vi "Dropable_DSA.vi"(0 "Analog In CH1":dbl, 1 "Cycle Specs":T3={"Cycles To Settle (M)"=5, "Cycles To Calculate (N)"=5}, 2 "Excitation Specs":T2={"Initial Frequency"=1.0, "Final Frequency"=100.0, "# of pts. in interval"=3, "Samping Time [s]"=0.001, "Amplitude [V]"=1.0, "Offset [V]"=0.5, "Freq Units (F: rad/s, T: Hz)"=FALSE}, 5 "Analog In CH0":dbl, 9 "START":bool, 11 "STOP":bool, 12 "Exit Porgram":bool) -> (4 "Analog Out":dbl, 6 "Bode Magnitude":cluster{dbl[], dbl[]}(graph)={[1.0, 1.2689610031679222, 1.6102620275609394, 2.043359717856942, 2.592943797404667, 3.2903445623126686, 4.1753189365604015, 5.298316906283708, 6.7233575364993365, 8.531678524172808, 10.826367338740546, 13.73823795883263, 17.43328822199988, 22.122162910704493, 28.072162039411772, 35.62247890262442, 45.20353656360243, 57.36152510448679, 72.7895384398315, 92.36708571873861, 117.21022975334806, 148.73521072935117, 188.73918221350976, 239.5026619987486, 303.9195382313198, 385.6620421163472, 489.3900918477494, 621.0169418915616, 788.0462815669912, 1000.0], [1.0018651131002922, 1.0016050465725763, 1.0010062349698785, 1.0002931137870483, 0.9991459144089636, 0.9972202532472595, 0.9944020144562293, 0.9903082002861369, 0.983855401702225, 0.9738705481650444, 0.9582906977613652, 0.9358034848813956, 0.9036393454169751, 0.857649976648417, 0.7964400088413218, 0.7217565791716765, 0.6359239660806931, 0.5476382842843324, 0.461415834347026, 0.38116988425483045, 0.3091314427820101, 0.2514928062528439, 0.20170891904461263, 0.15879614847289658, 0.127858110424497, 0.10171304349328705, 0.08081117825531599, 0.06376794604720305, 0.050469140870365095, 0.039745706120179934]}, 8 "Bode Phase":cluster{dbl[], dbl[]}(graph)={[1.0, 1.2689610031679222, 1.6102620275609394, 2.043359717856942, 2.592943797404667, 3.2903445623126686, 4.1753189365604015, 5.298316906283708, 6.7233575364993365, 8.531678524172808, 10.826367338740546, 13.73823795883263, 17.43328822199988, 22.122162910704493, 28.072162039411772, 35.62247890262442, 45.20353656360243, 57.36152510448679, 72.7895384398315, 92.36708571873861, 117.21022975334806, 148.73521072935117, 188.73918221350976, 239.5026619987486, 303.9195382313198, 385.6620421163472, 489.3900918477494, 621.0169418915616, 788.0462815669912, 1000.0], [-1.4001864556390353, -1.7425257743205063, -2.2774811113746067, -2.940300047591337, -3.797024621582645, -4.874740361894845, -6.244214499985965, -7.9488896703659435, -10.107416371370137, -12.8129960492024, -16.195047872218314, -20.2121008365249, -24.982209581081694, -30.62002310970157, -36.70295501035055, -43.18506539585506, -49.773026506300724, -56.0120451118291, -61.68921924132383, -66.61507141784128, -71.21117465500357, -75.07757805867544, -77.49128997241446, -81.82799122918105, -82.40583459630555, -84.09391534817092, -87.5421411007668, -88.23137376055858, -91.93060722680163, -98.46625820370649]}, 10 "Live signals":T1(graph), 14 "Stopped":bool, 15 "Running":bool)   [LabVIEW 2018]
doc: "Evaluate frequency response: CH1/CH0\n\nThis program performs 3 tasks:\n\n A.) generates a swept sine wave over a specified number of logmartically spaced frequencies over a specified range,\n\n B.) outputs the swept sine wave point by point to a system and for each point output measues the system's response at two points\n\n C.) and using the two responses measured, calculates the bode magnitude and phase plots between the two points of the system.\n\nThis program is written as a state machine that itterates one time for every iteration of the loop that contains it.\n \nThe state is the current sample being measured. \nNOTE: Since we must excite the system before recording data, the current sample being measured is one less than the number of itterations the loop containing this subVI has run.\n\nTo perform these tasks, the following state machine does the following:\n\n INITIALIZATION \n\n When initalized, the state is set to 0 and the following are calculated:\n\n A.) a list of logmartically spaced frequencies to excite the system at, \n B.) the number of samples needed to be ignored in waiting for the excitation to settle for each frequency, \n C.) the number of samples needed to be measured in order to calculate the frequency response for each frequency,\n D.) and the total number of samples needed (total # of smaples ignored + total # of samples measured).\n\n < see (1) INITIALIZE THE DSA section in the block diagram >\n\n RUNNING\n\n When running, the following tasks are done:\n\n A.) The swept sine wave for the next sample to be measured is generated and output. \n This is done by generating:\n\n 1.) the ith point of the swept sine wave to excite the system\n 2.) the frequency of the sine wave for the current point\n 3.) and the index of the frequency within the list excitation frequencies that corresponds to the i+1 point's sine wave's frequency.\n\n < see (2A) GENERATE SWEPT SINE EXCITATIONS section in the block diagram >\n\n B.) Compare the current sample to:\n\n 1.) the current last sample to be ignored in the list of last samples to be ignored\n 2.) and the current last smaple taken before chaning frequencies in the list of sample taken before the frequency change.\n\n < see (2B) COLLECT DATA? section in the block diagram >\n\n C.) If the current sample:\n \n 1.) < the current last sample to be ignored:\n \n - do nothing.\n \n 2.) = the current last sample to be ignored and:\n\n\n a.) < the current sample taken before changing frequencies:\n \n - collect a sample on each channel and store it\n\n < see (2C) ANALYZE DATA section in the block diagram >\n\n b.) = the current sample taken before changing frequencies:\n\n i.) collect a sample on each channel and store it,\n ii.) with all the other samples stored for that excitation frequency, calculate the magnitude and phase for each channel,\n iii.) use the magnitude and phase for each channel to calculate the magnitude and phase between the two points in the system,\n iv.) and plot the magnitude and phase between those two points in the system on the bode plot for the frequency.\n \n < see (2D) VERIFY DATA & (2E) PLOT section in the block diagram >\n\nInputs: \n\n- Excitation Specs:\n\n - Initial Frequency: The lowest frequency of the frequency range which the DSA will measure the bode plot for. \n\n - Final Frequency: The highest frequency of the frequency range which the DSA will measure the bode plot for. \n\n - Frequency Units: Whether the frequecny range input is in Hz or rads/sec. \n \n - Number of Frequencies: The number of logmarithmically spaced frequencies to measure the bode plot for.\n\n - Sampling Time: The time step taking in between each measurement. Also equal to 1/(sampling rate)\n\n - Amplitude: Amplitude of desired swept sine excitation. \n\n - Offset: DC offset of swept sine excitation.\n\n- Cycle Specs:\n\n - Cycles to Settle: The number of cycles of the swept sine wave at each frequency to ignore to let the transcient response die out. \n\n - Cycles to Calculate: The number of cycles of the sept since wave at each frequency to measure in order to measure the bode plot.\n\n- Controls:\n\n - START: Tells the DSA to initalize and then start.\n\n - STOP: Tells the DSA to stop and set all analog outputs to zero.\n\n - EXIT PROGRAM: Tells LabVIEW to set all analog outputs to zero and exit the program.\n\n- Signals:\n\n - Analog In CH1: Response read by the A/D converter of the system at a given point to the swept sine excitation.\n\n - Analog In CH0: Response read by the A/D converter of the system at a given point to the swept sine excitation.\n\nOutputs:\n\n- Analog Out: Swept sine excitation wave sent to the D/A converter.\n\n- Running: Signal to show if the DSA is running.\n\n- Stopped: Signal to show if the DSA is stopped.\n\n- Bode Magnitude: The magnitude plot of the TF CH1/CH0.\n\n- Bode Phase: The phase plot of the TF CH1/CH0."
panel:
  # "Dropable Dynamic Signal Analyzer"
  # "Magnitude"
  # "Dynamic Signal Analyzer"
  # "Controls"
  # "Signals"
  # "Phase"
  # "Excitation Frequencies"
  # "Frequency\nUnits"
  # "[Hz]"
  # "Excitation Magnitude"
  # "[rad/s]"
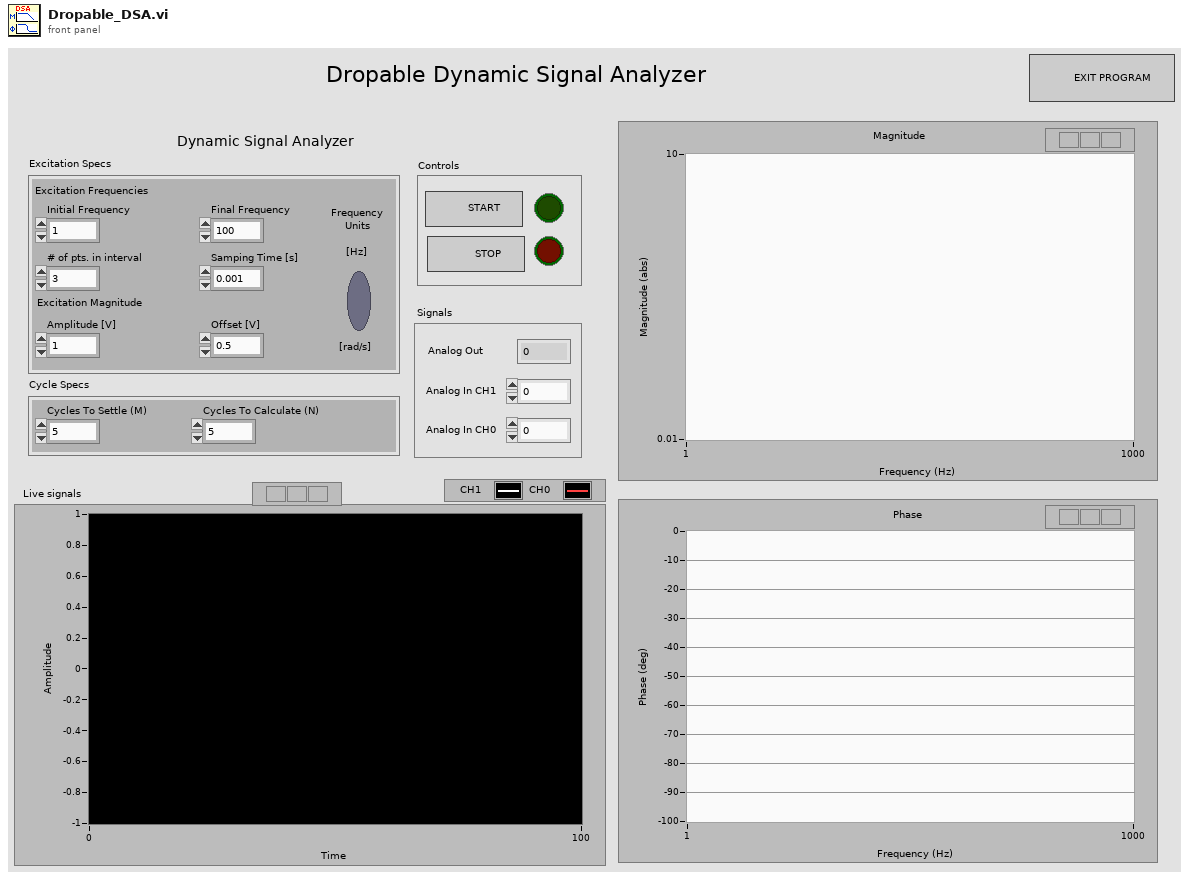
[diagram p1: front panel]
types:
  T1 = cluster{"Analog In CH1":dbl, "Analog In CH0":dbl}
  T2 = cluster{"Initial Frequency":dbl, "Final Frequency":dbl, "# of pts. in interval":i16, "Samping Time [s]":dbl, "Amplitude [V]":dbl, "Offset [V]":dbl, "Freq Units (F: rad/s, T: Hz)":bool}
  T3 = cluster{"Cycles To Settle (M)":i16, "Cycles To Calculate (N)":i16}
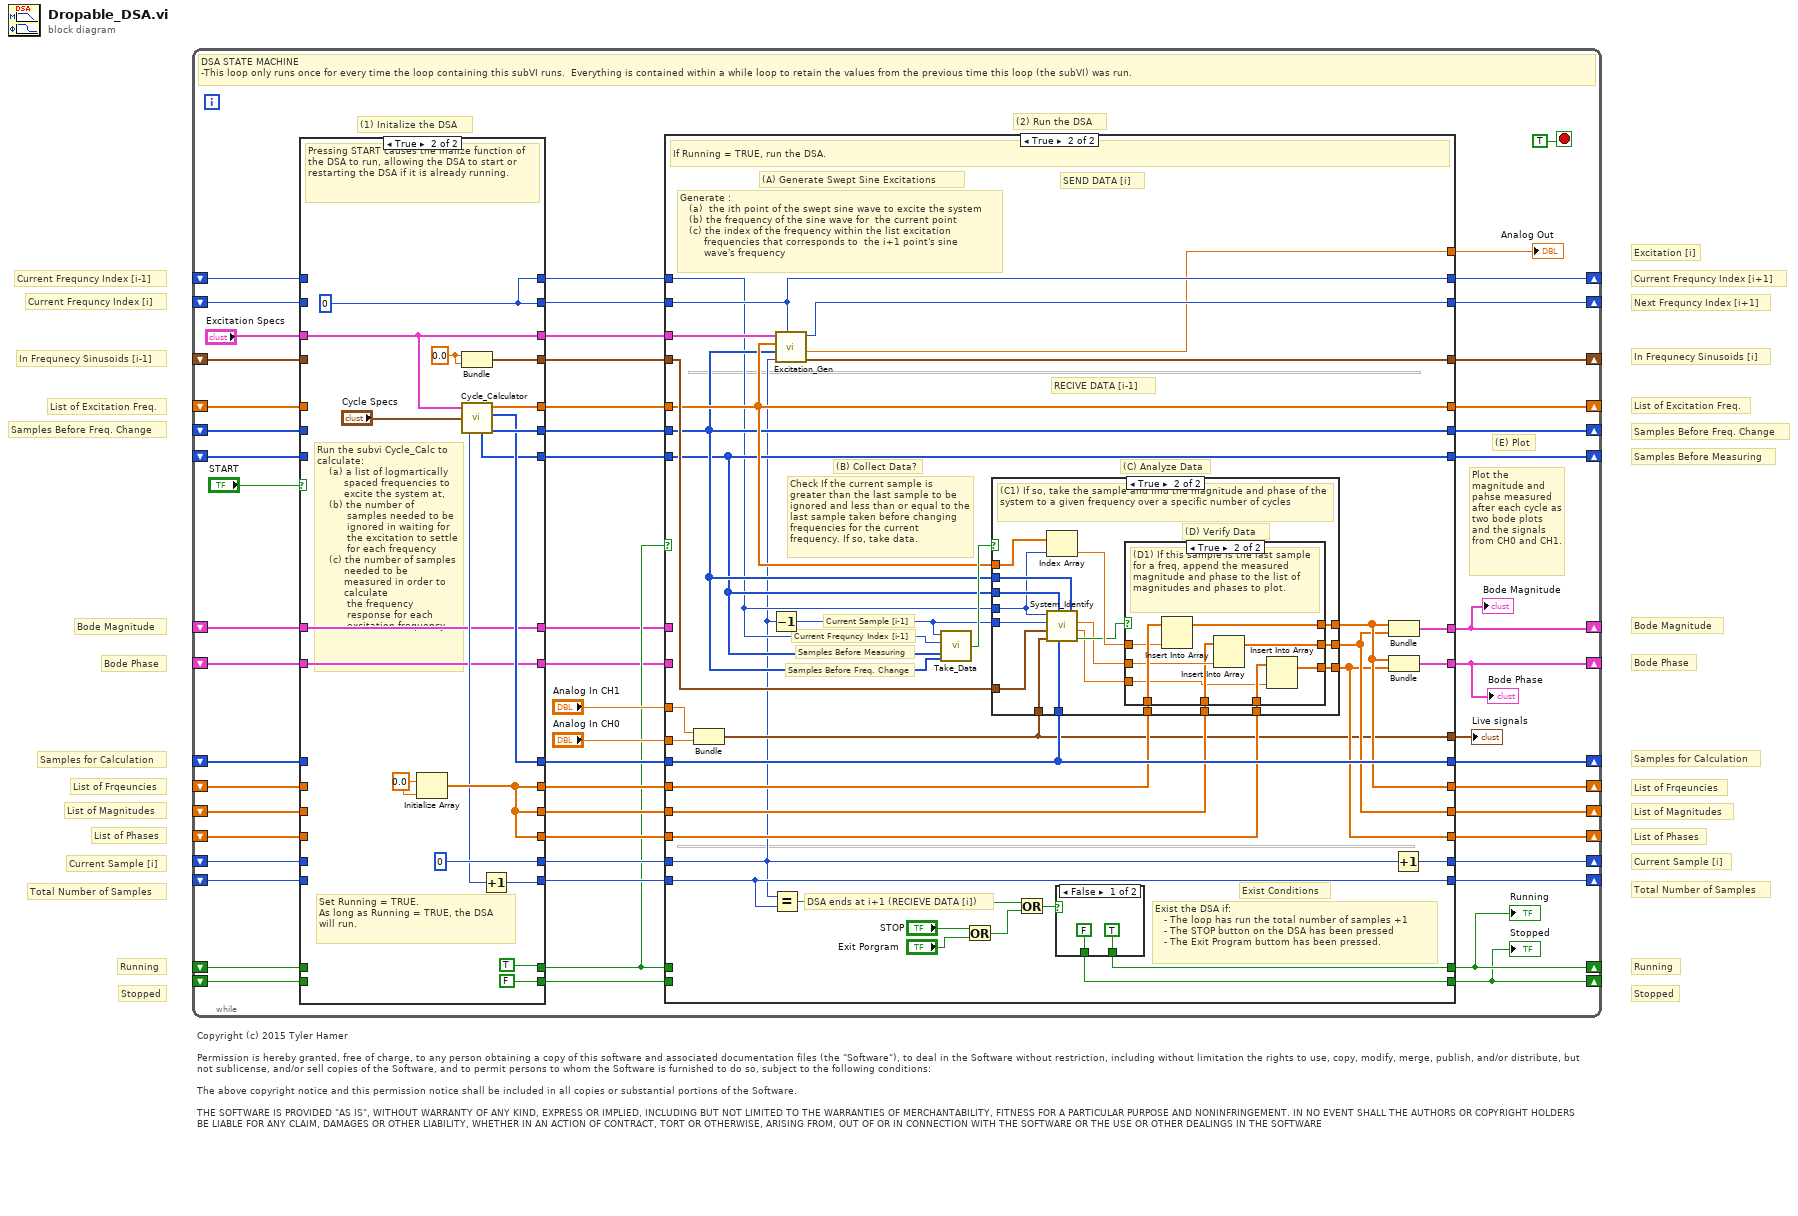
[diagram p0: block diagram]
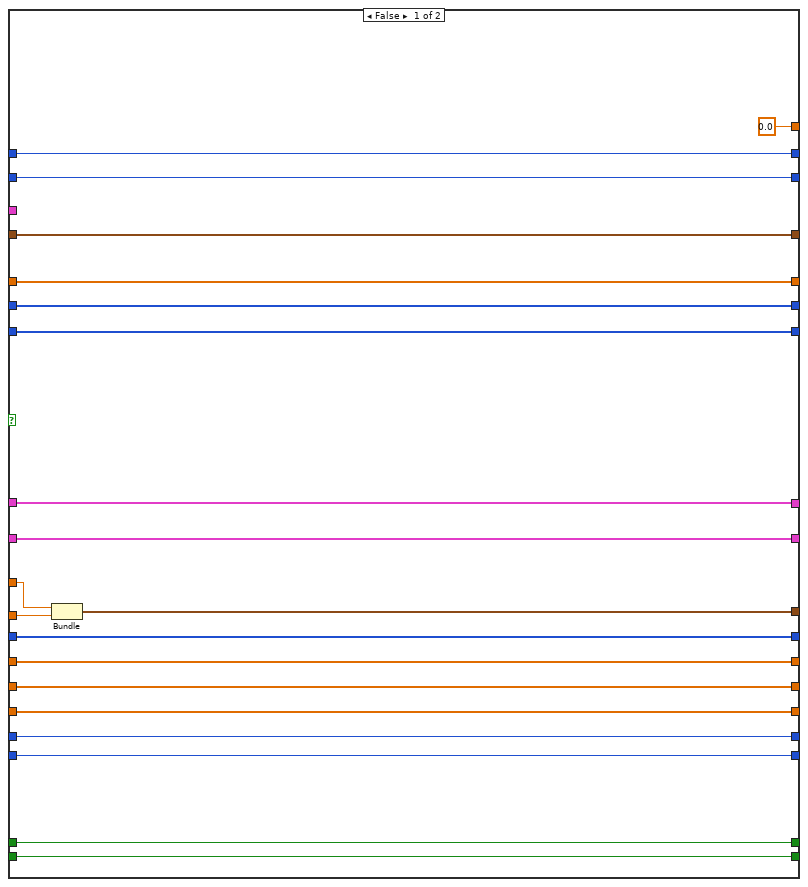
[diagram p2: hidden frame]
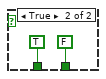
[diagram p3: hidden frame]
diagram:
  # "Copyright (c) 2015 Tyler Hamer\n\nPermission is hereby granted, free of charge, to any person obtaining a copy of this software and associated documentation files (the \"Software\"), to deal in the Software without restriction, including without limitation the rights to use, copy, modify, merge, publish, and/or distribute, but not sublicense, and/or sell copies of the Software, and to permit persons to whom the Software is furnished to do so, subject to the following conditions:\n\nThe above copyright notice and this permission notice shall be included in all copies or substantial portions of the Software.\n\nTHE SOFTWARE IS PROVIDED \"AS IS\", WITHOUT WARRANTY OF ANY KIND, EXPRESS OR IMPLIED, INCLUDING BUT NOT LIMITED TO THE WARRANTIES OF MERCHANTABILITY, FITNESS FOR A PARTICULAR PURPOSE AND NONINFRINGEMENT. IN NO EVENT SHALL THE AUTHORS OR COPYRIGHT HOLDERS BE LIABLE FOR ANY CLAIM, DAMAGES OR OTHER LIABILITY, WHETHER IN AN ACTION OF CONTRACT, TORT OR OTHERWISE, ARISING FROM, OUT OF OR IN CONNECTION WITH THE SOFTWARE OR THE USE OR OTHER DEALINGS IN THE SOFTWARE"
  # "Bode Phase"
  # "Bode Magnitude"
  # "Bode Phase"
  # "Bode Magnitude"
  # "Stopped"
  # "Running"
  # "Stopped"
  # "Running"
  # "Total Number of Samples"
  # "Total Number of Samples"
  # "List of Phases"
  # "List of Magnitudes"
  # "List of Frqeuncies"
  # "List of Phases"
  # "List of Magnitudes"
  # "List of Frqeuncies"
  # "Samples Before Measuring"
  # "Samples Before Freq. Change"
  # "Current Sample [i]"
  # "Samples for Calculation"
  # "Excitation [i]"
  # "List of Excitation Freq."
  # "In Frequnecy Sinusoids [i]"
  # "Next Frequncy Index [i+1]"
  # "Current Frequncy Index [i+1]"
  # "Samples for Calculation"
  # "Current Sample [i]"
  # "Samples Before Freq. Change"
  # "In Frequnecy Sinusoids [i-1]"
  # "Current Frequncy Index [i-1]"
  # "Current Frequncy Index [i]"
  # "List of Excitation Freq."
  n1 = while {
    shift-right: [w48] -> _
    shift-left: _ -> [w52]
    shift-right: [w50] -> _
    shift-left: _ -> [w51]
    shift-right: [w46] -> _
    shift-left: _ -> [w45]
    shift-right: [w39] -> _
    shift-left: _ -> [w49]
    shift-right: [w43] -> _
    shift-left: _ -> [w42]
    shift-right: [w36] -> _
    shift-left: _ -> [w35]
    shift-right: [w33] -> _
    shift-left: _ -> [w32]
    shift-right: [w30] -> _
    shift-left: _ -> [w29]
    shift-right: [w20] -> _
    shift-left: _ -> [w23]
    shift-right: [w19] -> _
    shift-left: _ -> [w22]
    shift-right: [w18] -> _
    shift-left: _ -> [w21]
    shift-right: [w15] -> _
    shift-left: _ -> [w14]
    shift-right: [w9] -> _
    shift-left: _ -> [w13]
    shift-right: [w8] -> _
    shift-left: _ -> [w10]
    shift-right: [w3] -> _
    shift-left: _ -> [w7]
    shift-right: [w2] -> _
    shift-left: _ -> [w6]
    stop <- TRUE stop-if-true
    # "Plot the magnitude and pahse measured after each cycle as two bode plots and the signals from CH0 and CH1."
    # "(E) Plot"
    # "(2) Run the DSA"
    # "(1) Initalize the DSA"
    # "DSA STATE MACHINE \n-This loop only runs once for every time the loop containing this subVI runs.  Everything is contained within a while loop to retain the values from the previous time this loop (the subVI) was run."
    n2 = case shown="True" "START" {
      tunnel: "Excitation Specs" -> [w164 w181]
      tunnel: [w164 w181] -> w54
      tunnel: [w162 w180] -> w53
      tunnel: w52 -> [w162 _]
      tunnel: [w163 w178] -> w47
      tunnel: w51 -> [w163 _]
      tunnel: [w159 w179] -> w40
      tunnel: w49 -> [w159 _]
      tunnel: [w161 w178] -> w44
      tunnel: w45 -> [w161 _]
      tunnel: w42 -> [w160 _]
      tunnel: [w160 w176] -> w41
      tunnel: [w158 0] -> w38
      tunnel: w35 -> [w158 _]
      tunnel: [w157 w174] -> w34
      tunnel: w32 -> [w157 _]
      tunnel: [w156 w173] -> w31
      tunnel: w29 -> [w156 _]
      tunnel: [w155 w171] -> w26
      tunnel: [w154 w171] -> w25
      tunnel: [w153 w171] -> w24
      tunnel: w23 -> [w155 _]
      tunnel: w22 -> [w154 _]
      tunnel: w21 -> [w153 _]
      tunnel: [w152 w168] -> w16
      tunnel: w14 -> [w152 _]
      tunnel: w13 -> [w151 _]
      tunnel: [w151 TRUE] -> w12
      tunnel: [w150 FALSE] -> w11
      tunnel: w10 -> [w150 _]
      tunnel: w7 -> [w149 w166]
      tunnel: w6 -> [w148 w165]
      tunnel: [w149 w166] -> w5
      tunnel: [w148 w165] -> w4
      frame False {
      }
      frame True {
        w172 = 0.0
        w177 = 0.0
        w178 = 0
        # "Run the subvi Cycle_Calc to calculate: \n    (a) a list of logmartically \n         spaced frequencies to \n         excite the system at, \n    (b) the number of \n          samples needed to be \n          ignored in waiting for \n          the excitation to settle \n          for each frequency \n    (c) the number of samples \n         needed to be \n         measured in order to\n         calculate \n          the frequency   \n          response for each \n          excitation frequency."
        # "Set Running = TRUE.\nAs long as Running = TRUE, the DSA\nwill run."
        # "Pressing START causes the inalize function of the DSA to run, allowing the DSA to start or restarting the DSA if it is already running."
        n3 = Initialize Array(w172, w172) -> (w171:dbl[])
        n4 = Bundle(w177, w177) -> (w176:cluster{dbl, dbl})  [unwired: 1 in]
        n5 = call "Cycle_Calculator.vi"("Cycle Specs"="Cycle Specs", "Excitation Specs"=w181) -> ("Samples Before Frequency Change"=w179:i32[], "Samples Before Measuring"=w173:i32[], "Samples for Calculation"=w174:i32[], "Excitation Frequencies"=w180:dbl[], "Total Number of Samples"=w167:i32)  [unwired: 1 in, 1 out]
        n6 = Increment(x=w167) -> (x+1=w168:i32)
      }
    }
    n7 = case shown="True" w12 {
      tunnel: w54 -> [_ w110]
      tunnel: w53 -> [w76 w103]
      tunnel: [w75 w109] -> w50
      tunnel: [w76 w103] -> w48
      tunnel: w47 -> [w75 w108]
      tunnel: [w74 w108] -> w46
      tunnel: w44 -> [w74 w100]
      tunnel: [w73 w107] -> w43
      tunnel: w41 -> [w73 w104]
      tunnel: w40 -> [w72 w102]
      tunnel: [w72 w102] -> w39
      tunnel: w38 -> [w71 w77]
      tunnel: [w71 w106] -> w36
      tunnel: w34 -> [w70 w96]
      tunnel: [w70 w96] -> w33
      tunnel: w31 -> [w69 w101]
      tunnel: [w69 w101] -> w30
      tunnel: "Analog In CH1" -> [w60 w98]
      tunnel: "Analog In CH0" -> [w59 w97]
      tunnel: w26 -> [w68 w95]
      tunnel: w25 -> [w67 w94]
      tunnel: w24 -> [w66 w93]
      tunnel: [w68 w92] -> w20
      tunnel: [w67 w91] -> w19
      tunnel: [w66 w90] -> w18
      tunnel: [0.0 w89] -> w17
      tunnel: w16 -> [w65 w81]
      tunnel: [w65 w81] -> w15
      tunnel: w12 -> [w64 _]
      tunnel: [w64 w83] -> w9
      tunnel: [w63 w82] -> w8
      tunnel: w11 -> [w63 _]
      tunnel: [w62 w79] -> w3
      tunnel: [w61 w78] -> w2
      tunnel: w5 -> [w62 _]
      tunnel: w4 -> [w61 _]
      tunnel: [w58 w80] -> w1
      frame False {
        n8 = Bundle("Analog In CH1"=w60, "Analog In CH0"=w59) -> (w58:T1)  [unwired: 1 in]
      }
      frame True {
        # "(C) Analyze Data"
        # "Exist Conditions"
        # "Exist the DSA if:\n   - The loop has run the total number of samples +1\n   - The STOP button on the DSA has been pressed\n   - The Exit Program buttom has been pressed."
        # "DSA ends at i+1 (RECIEVE DATA [i])"
        # "SEND DATA [i]"
        # "RECIVE DATA [i-1]"
        # "Samples Before Freq. Change"
        # "Samples Before Measuring"
        # "Current Frequncy Index [i-1]"
        # "Current Sample [i-1]"
        # "(B) Collect Data?"
        # "Check If the current sample is greater than the last sample to be ignored and less than or equal to the last sample taken before changing frequencies for the current frequency. If so, take data."
        # "(A) Generate Swept Sine Excitations"
        # "Generate :\n   (a)  the ith point of the swept sine wave to excite the system\n   (b) the frequency of the sine wave for  the current point\n   (c) the index of the frequency within the list excitation \n        frequencies that corresponds to  the i+1 point's sine \n        wave's frequency"
        # "If Running = TRUE, run the DSA."
        n9 = Bundle("Analog In CH1"=w98, "Analog In CH0"=w97) -> (w80:T1)  [unwired: 1 in]
        n10 = Decrement(x=w77) -> (x-1=w99:i32)
        n11 = Equal?(x=w77, y=w81) -> (x = y?=w88:bool)
        n12 = call "Excitation_Gen.vi"("Current Frequency Index"=w108, "Current Sample"=w77, "Samples Before Frequency Change"=w102, "Excitation Frequencies"=w103, "Excitation Specs"=w110) -> ("In Frequency Sinusoids"=w107:cluster{"cos(wt)":dbl, " sin(wt)":dbl}, "Excitation Sinusoid"=w89:dbl, "New Frequency Index"=w109:i32)  [unwired: 1 out]
        n13 = call "Take_Data.vi"("Samples Before Frequency Change"=w102, "Samples Before Measuring"=w101, "Current Frequency Index"=w100, "Current Sample"=w99) -> ("Take Data"=w105:bool)
        n14 = Or(x="STOP", y="Exit Porgram") -> (x .or. y?=w85:bool)
        n15 = case shown="True" w105 {
          tunnel: w104 -> [_ w131]
          tunnel: w80 -> [_ w135]
          tunnel: w99 -> [_ w134]
          tunnel: w100 -> [_ w128]
          tunnel: w101 -> [_ w133]
          tunnel: w102 -> [_ w132]
          tunnel: w103 -> [_ w130]
          tunnel: w96 -> [_ w129]
          tunnel: w95 -> [w117 w123]
          tunnel: w94 -> [w116 w122]
          tunnel: w93 -> [w115 w121]
          tunnel: [w117 w120] -> w92
          tunnel: [w116 w119] -> w91
          tunnel: [w115 w118] -> w90
          frame False {
            # "(C2) If not, ignore the current samples. Pass throught the list of measured magnitude and phases though."
          }
          frame True {
            # "(D) Verify Data"
            # "(C1) If so, take the sample and find the magnitude and phase of the system to a given frequency over a specific number of cycles"
            n16 = Index Array(array=w130, index=w128) -> (element=w127:dbl)
            n17 = call "System_Identify.vi"("Samples Before Frequency Change"=w132, "Samples for Calculation"=w129, "Samples Before Measuring"=w133, "Frequency Responses"=w135, "In Frequency Sinusoids"=w131, "Current Sample"=w134, "Current Frequency Index"=w128) -> ("Push To Plot"=w126:bool, "System Phase"=w124:dbl, "System Magnitude"=w125:dbl)
            n18 = case shown="True" w126 {
              tunnel: w127 -> [_ w146]
              tunnel: w125 -> [_ w145]
              tunnel: w124 -> [_ w142]
              tunnel: w123 -> [w138 w147]
              tunnel: w122 -> [w137 w144]
              tunnel: w121 -> [w136 w143]
              tunnel: [w138 w141] -> w120
              tunnel: [w137 w140] -> w119
              tunnel: [w136 w139] -> w118
              frame False {
                # "(D2) If this sample is not the last sample for a freq, the current measured magnitude and phase are not accurate yet."
              }
              frame True {
                # "(D1) If this sample is the last sample for a freq, append the measured magnitude and phase to the list of magnitudes and phases to plot."
                n19 = Insert Into Array(array=w147, new element=w146) -> (w141:dbl[])  [unwired: 1 in]
                n20 = Insert Into Array(array=w144, new element=w145) -> (w140:dbl[])  [unwired: 1 in]
                n21 = Insert Into Array(array=w143, new element=w142) -> (w139:dbl[])  [unwired: 1 in]
              }
            }
          }
        }
        n22 = Or(x=w88, y=w85) -> (x .or. y?=w84:bool)
        n23 = case shown="False" w84 {
          tunnel: [TRUE FALSE] -> w83
          tunnel: [FALSE TRUE] -> w82
          frame False {
          }
          frame True {
          }
        }
        n24 = Bundle(w92, w91) -> (w79:cluster{dbl[], dbl[]})  [unwired: 1 in]
        n25 = Bundle(w92, w90) -> (w78:cluster{dbl[], dbl[]})  [unwired: 1 in]
        n26 = Increment(x=w77) -> (x+1=w106:i32)
      }
    }
    "Analog Out" <- w17
    "Running" <- w9
    "Stopped" <- w8
    "Bode Magnitude" <- w3
    "Bode Phase" <- w2
    "Live signals" <- w1
  }
